vi "Kernel - FPGA Data Acquisition.vi"(7 "Data in - FPGA Data Acquisition":T1={"Count (uSec)"=0, "Timed Out?"=FALSE, "Samples per Channel"=2000}, 8 "error in":errorcluster, 10 "State":string, 11 "message queue":refnum<queue>) -> (0 "error out":errorcluster, 3 "message queue (out)":refnum<queue>, 4 "Stop?":bool, 5 "Data out - FPGA Data Acquisition":T1={"Count (uSec)"=0, "Timed Out?"=FALSE, "Samples per Channel"=2000})   [LabVIEW 2021]
uses:
  Typedefs/Data - FPGA Data Acquisition.ctl
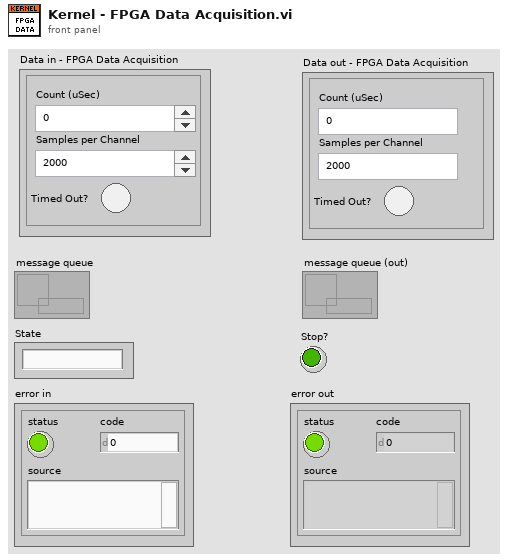
[diagram p1: front panel]
types:
  T1 = typedef "Data - FPGA Data Acquisition.ctl" = cluster{"Count (uSec)":i32, "Timed Out?":bool, "Samples per Channel":i32}
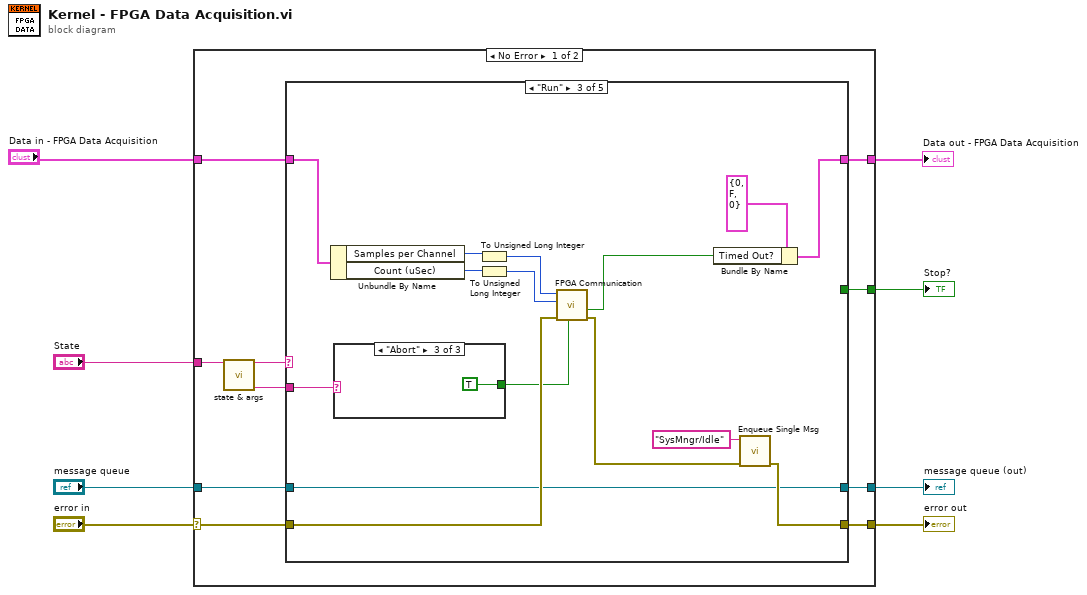
[diagram p0: block diagram]
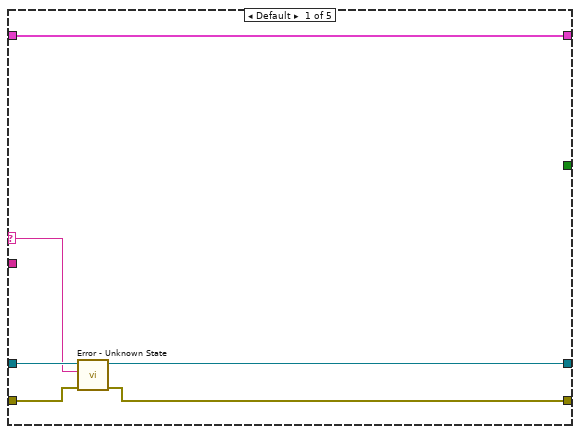
[diagram p2: hidden frame]
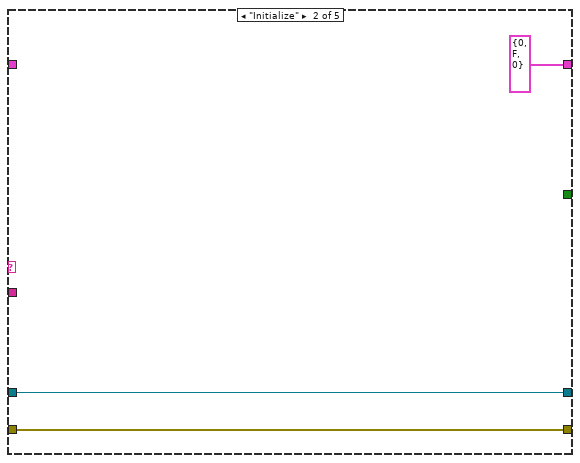
[diagram p3: hidden frame]
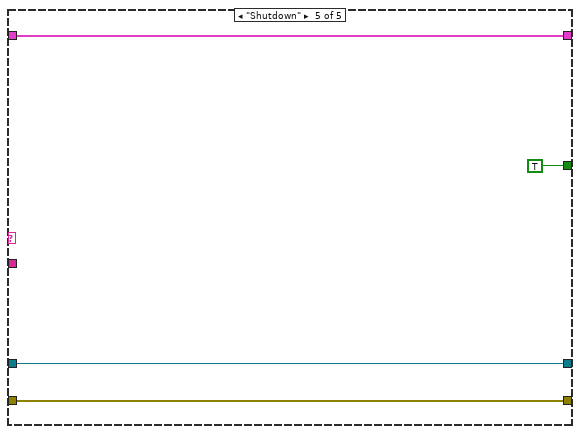
[diagram p7: hidden frame]
diagram:
  n1 = case shown="No Error" "error in" {
    selector: "error in" -> [w14 w52]
    tunnel: "State" -> [w18 _]
    tunnel: "message queue" -> [w15 w53]
    tunnel: [w13 w53] -> w5
    tunnel: [w12 w52] -> w4
    tunnel: [w11 _] -> w3
    tunnel: [w10 w51] -> w2
    tunnel: "Data in - FPGA Data Acquisition" -> [w9 w51]
    frame No Error {
      n2 = call "state & args.vi"("state:args"=w18) -> ("args"=w16:string, "state"=w17:string)  [unwired: 9 in]
      n3 = case shown="\"Run\"" w17 {
        selector: w17 -> [w22 _ _ _ _]
        tunnel: w16 -> [_ _ w33 _ _]
        tunnel: w15 -> [w24 w27 w28 w45 w49]
        tunnel: w14 -> [w23 w25 w42 w44 w48]
        tunnel: [w21 w27 w28 w45 w49] -> w13
        tunnel: [w20 w25 w29 w44 w48] -> w12
        tunnel: [_ _ _ _ TRUE] -> w11
        tunnel: [w19 T1 {"Count (uSec)"=0, "Timed Out?"=FALSE, "Samples per Channel"=0} ("Data in - FPGA Data Acquisition") w34 w46 w47] -> w10
        tunnel: w9 -> [w19 _ w41 w46 w47]
        frame Default {
          n4 = call "Error - Unknown State.vi"("error in"=w23, "state"=w22, "queue"=w24) -> ("error out"=w20:errorcluster, "queue out"=w21:refnum<queue>)  [unwired: 7 in]
        }
        frame "Initialize" {
        }
        frame "Run" {
          n5 = Unbundle By Name(w41) -> ("Samples per Channel"=w40:i32, "Count (uSec)"=w39:i32)
          n6 = case shown="\"Abort\"" w33 {
            tunnel: [_ _ TRUE] -> w32
            frame "False" {
            }
            frame Default {
            }
            frame "Abort" {
            }
          }
          n7 = To Unsigned Long Integer(number=w40) -> (unsigned 32bit integer=w38:u32)
          n8 = To Unsigned Long Integer(number=w39) -> (unsigned 32bit integer=w37:u32)
          n9 = call "FPGA Communication.vi"("Stop Button"=w32, "error in"=w42, "Count(uSec)"=w37, "Samples per Channel"=w38) -> ("error out"=w30:errorcluster, "Timed Out?"=w35:bool)  [unwired: 6 in]
          n10 = Bundle By Name(cluster=T1 {"Count (uSec)"=0, "Timed Out?"=FALSE, "Samples per Channel"=0} ("Data in - FPGA Data Acquisition"), "Timed Out?"=w35) -> (w34:T1)
          n11 = call "Enqueue Single Msg.vi"("error in"=w30, "queue/message"="SysMngr/Idle") -> ("error out"=w29:errorcluster)  [unwired: 9 in]
        }
        frame "Error" {
        }
        frame "Shutdown" {
        }
      }
    }
    frame Error {
    }
  }
  "error out" <- w4
  "Stop?" <- w3
  "message queue (out)" <- w5
  "Data out - FPGA Data Acquisition" <- w2
